vi "Global.vi"() -> ()   [LabVIEW 2016]
panel:
  in  "UserGroup":string
  in  "UserName":string
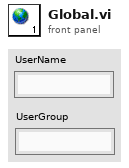
[diagram p1: front panel]
diagram:
